vi "Longest Line Length in Pixels.vi"(10 "String":refnum<vi>) -> (3 "longest line length":i32 caption="Längste Zeilenlänge")   [LabVIEW 2009]
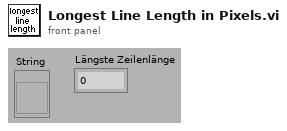
[diagram p1: front panel]
types:
  T1 = enum16{"User-specified Font", "Application Font", "System Font", "Dialog Font"}
  T2 = cluster{"horizontal":enum16{"left", "center", "right"}, "vertical":enum16{"top", "center", "bottom"}}
  T3 = typedef "LVFontTypeDef.ctl" = cluster{"Font Name":string, "Size":u16, "Bold":bool, "Italic":bool, "Underline":bool, "Strikeout":bool, "Color":u32}
  T4 = cluster{"Font Name:":string, "Size":i16, "Strikeout?":bool, "Italic?":bool, "Underline?":bool, "Outline?":bool, "Shadow?":bool, "Bold?":bool}
  T5 = cluster{"left":i16, "top":i16, "right":i16, "bottom":i16}
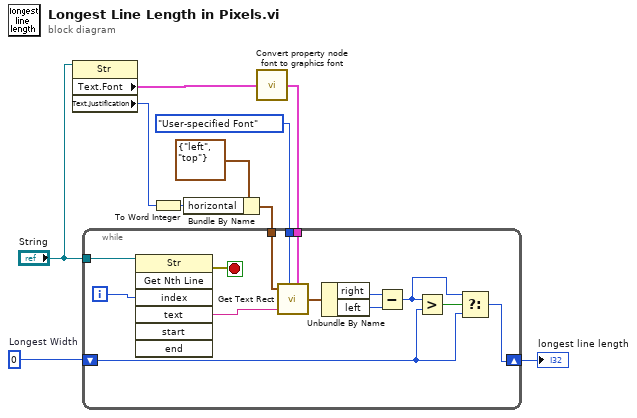
[diagram p0: block diagram]
diagram:
  w2 = 0  # Longest Width
  n1 = property class="Str"(reference="String") -> ("Text.Font"=w9:T3, "Text.Justification"=w5:enum16{"Left", "Center", "Right"})  [unwired: 1 in, 2 out]
  n2 = To Word Integer(number=w5) -> (16bit integer=w4:i16)
  n3 = Bundle By Name(cluster=T2 {"horizontal"=enum."left", "vertical"=enum."top"} ("alignment(left, top)"), "horizontal"=w4) -> (w7:T2)
  n4 = call "Convert property node font to graphics font.vi"("String:Text:Font:All Elements font cluster"=w9) -> ("Get Text Rect font cluster"=w8:T4)
  n5 = while {
    tunnel: "String" -> [w24]
    tunnel: w7 -> [w22]
    tunnel: w8 -> [w16]
    tunnel: T1."User-specified Font" ("desired font(Application)") -> [w15]
    shift-right: [w11] -> w1
    shift-left: w2 -> [w12]
    i -> [w18]
    stop <- w17 stop-if-true
    n6 = invoke class="Str" method="Get Nth Line"(reference=w24, "index"=w18) -> (error out=w17:errorcluster, "text"=w23:string)  [unwired: 5 in, 5 out]
    n7 = call <vilib>:"Get Text Rect.vi"("alignment(left, top)"=w22, "desired font(Application)"=w15, "text"=w23, "[user-specified font]"=w16) -> ("rect"=w21:T5)  [unwired: 5 in]
    n8 = Unbundle By Name(w21) -> ("right"=w19:i16, "left"=w20:i16)
    n9 = Subtract(x=w19, y=w20) -> (x-y=w13:i16)
    n10 = Greater?(x=w13, y=w12) -> (0:w14:bool)
    n11 = Select(t=w13, s=w14, f=w12) -> (s? t:f=w11:i32)
  }
  "longest line length" <- w1
